vi "VG_0Detected.vi"() -> ()   [LabVIEW 2020]
panel:
  out "0 Detected":bool
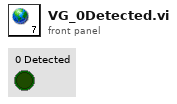
[diagram p1: front panel]
diagram:
